vi "SV Limit Testing for Monitoring (N Ch) (waveform) (DBL).vi"(7 "reset":bool, 9 "lower limit":dbl=-inf format="%.2f", 10 "upper limit":dbl=inf format="%.2f", 11 "input signals":waveform(dbl)[](array[waveform])) -> (1 "lower limit clearances":dbl[](array[numeric]) format="%.6f", 2 "upper limit clearances":dbl[](array[numeric]) format="%.6f", 3 "tests passed":bool[](array[boolean]), 5 "timestamps":timestamp[](array[timestamp]) format="%<%.6X\n%x>T")   [LabVIEW 2017]
doc: "Performs limit testing on waveforms, spectra, XY data, identified peaks, or scalar measurements. You can wire <B>output values</B> to a graph to view the limits, signal, and failures. Wire data to the<B> signal in</B> input to determine the polymorphic instance to use or manually select the instance."
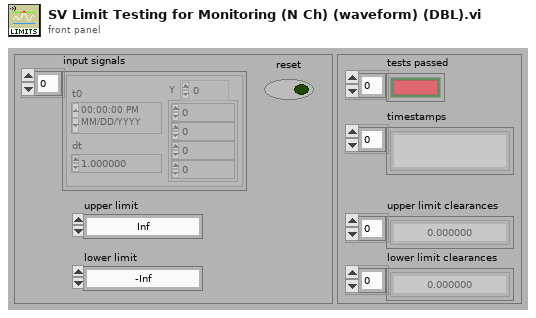
[diagram p1: front panel]
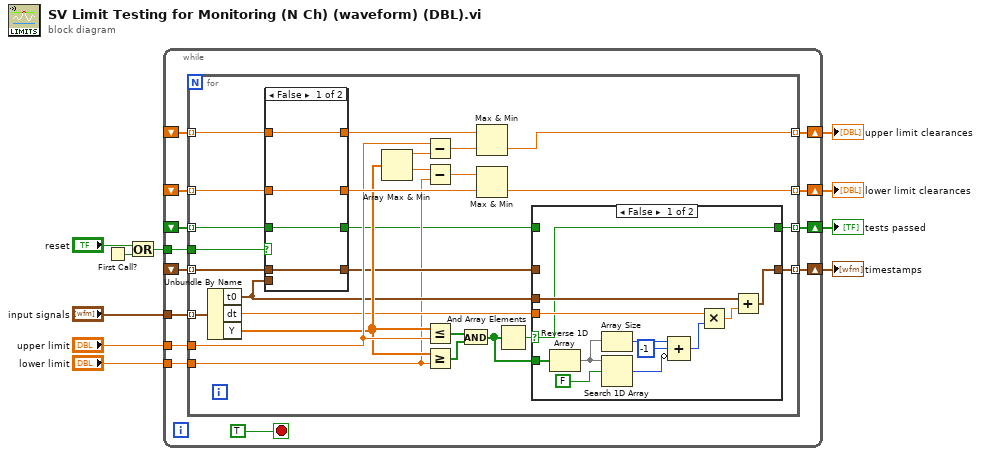
[diagram p0: block diagram]
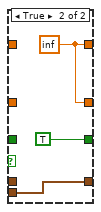
[diagram p3: hidden frame]
diagram:
  n1 = First Call?() -> (First Call?: T/F=w2:bool)
  n2 = Or(x="reset", y=w2) -> (x .or. y?=w3:bool)
  n3 = while {
    tunnel: "input signals" -> [w23]
    tunnel: "upper limit" -> [w15]
    tunnel: "lower limit" -> [w12]
    shift-right: [w22] -> w7
    shift-left: _ -> [w19]
    shift-right: [w21] -> w6
    shift-left: _ -> [w18]
    shift-right: [w11] -> w5
    shift-left: _ -> [w17]
    shift-right: [w14] -> w1
    shift-left: _ -> [w16]
    tunnel: w3 -> [w20]
    stop <- TRUE stop-if-true
    n4 = for {
      tunnel: w23 -> [w50] mode=indexing
      tunnel: [w49] -> w22 mode=indexing
      tunnel: [w48] -> w21 mode=indexing
      tunnel: w20 -> [w47]
      tunnel: w19 -> [w46] mode=indexing
      tunnel: w18 -> [w44] mode=indexing
      tunnel: w17 -> [w42] mode=indexing
      tunnel: w16 -> [w41] mode=indexing
      tunnel: w15 -> [w40]
      tunnel: [w36] -> w14 mode=indexing
      tunnel: w12 -> [w30]
      tunnel: [w28] -> w11 mode=indexing
      n5 = Unbundle By Name(w50) -> ("t0"=w35:timestamp, "dt"=w34:dbl, "Y"=w39:dbl[])
      n6 = case shown="False" w47 {
        tunnel: w46 -> [w68 _]
        tunnel: [w68 w69] -> w45
        tunnel: w44 -> [w67 _]
        tunnel: [w67 w69] -> w43
        tunnel: w42 -> [w66 _]
        tunnel: [w66 TRUE] -> w29
        tunnel: w41 -> [w65 _]
        tunnel: [w65 w71] -> w37
        tunnel: w35 -> [_ w71]
        frame False {
        }
        frame True {
          w69 = inf
        }
      }
      n7 = Array Max & Min(array=w39) -> (max value=w27:dbl, min value=w26:dbl)  [unwired: 2 out]
      n8 = Subtract(x=w40, y=w27) -> (x-y=w25:dbl)
      n9 = Subtract(x=w26, y=w30) -> (x-y=w24:dbl)
      n10 = Less Or Equal?(x=w39, y=w40) -> (x <= y?=w32:bool[])
      n11 = Greater Or Equal?(x=w39, y=w30) -> (x >= y?=w31:bool[])
      n12 = And(x=w32, y=w31) -> (x .and. y?=w38:bool[])
      n13 = Max & Min(x=w45, y=w25) -> (min(x,y)=w49:dbl)  [unwired: 1 out]
      n14 = Max & Min(x=w24, y=w43) -> (min(x,y)=w48:dbl)  [unwired: 1 out]
      n15 = And Array Elements(Boolean array=w38) -> (logical AND=w33:bool)
      n16 = case shown="False" w33 {
        selector: w33 -> [w51 _]
        tunnel: w38 -> [w61 _]
        tunnel: w37 -> [_ w64]
        tunnel: [w55 w64] -> w36
        tunnel: w35 -> [w56 _]
        tunnel: w34 -> [w52 _]
        tunnel: w29 -> [_ w63]
        tunnel: [w51 w63] -> w28
        frame False {
          n17 = Reverse 1D Array(array=w61) -> (reversed array=w60:bool[])
          n18 = Array Size(array=w60) -> (size(s)=w59:i32)
          n19 = Search 1D Array(1D array=w60, element=FALSE) -> (index of element=w57:i32)  [unwired: 1 in]
          n20 = Compound Arithmetic op=ADD(w59, -1 ("value"), invert w57) -> (w53:i32)
          n21 = Multiply(x=w52, y=w53) -> (x*y=w54:dbl)
          n22 = Add(x=w56, y=w54) -> (x+y=w55:timestamp)
        }
        frame True {
        }
      }
    }
  }
  "tests passed" <- w5
  "upper limit clearances" <- w7
  "lower limit clearances" <- w6
  "timestamps" <- w1
